vi "25-1.vi"() -> ()   [LabVIEW 2019, in "25.lvlib"]
uses:
  25.lvlib
panel:
  in  "Sample?":bool
  out "Array":u32[][](array[colorbox])
  out "Steps":i32
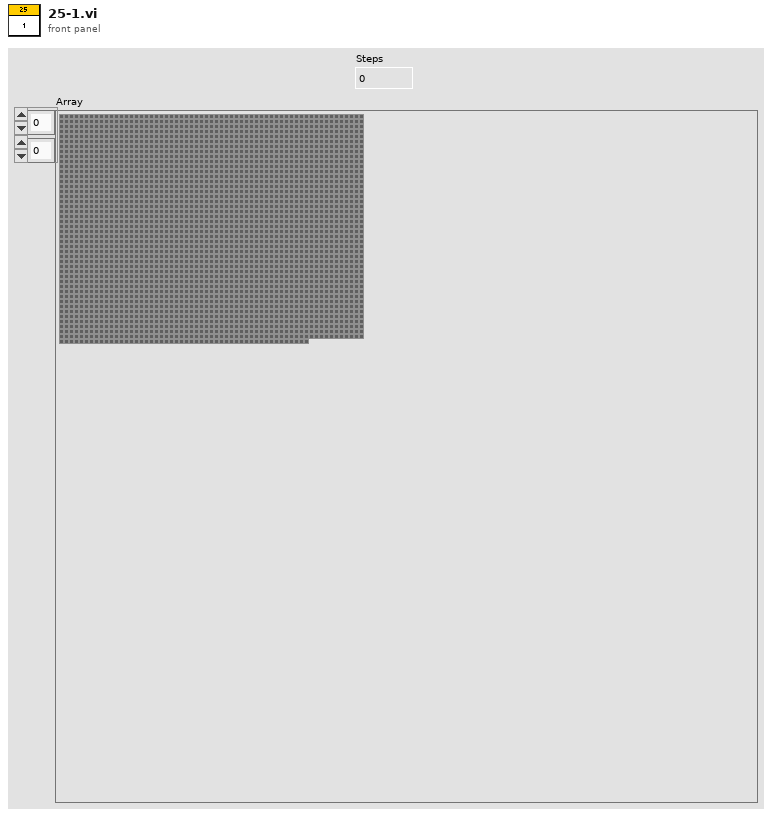
[diagram p1: front panel]
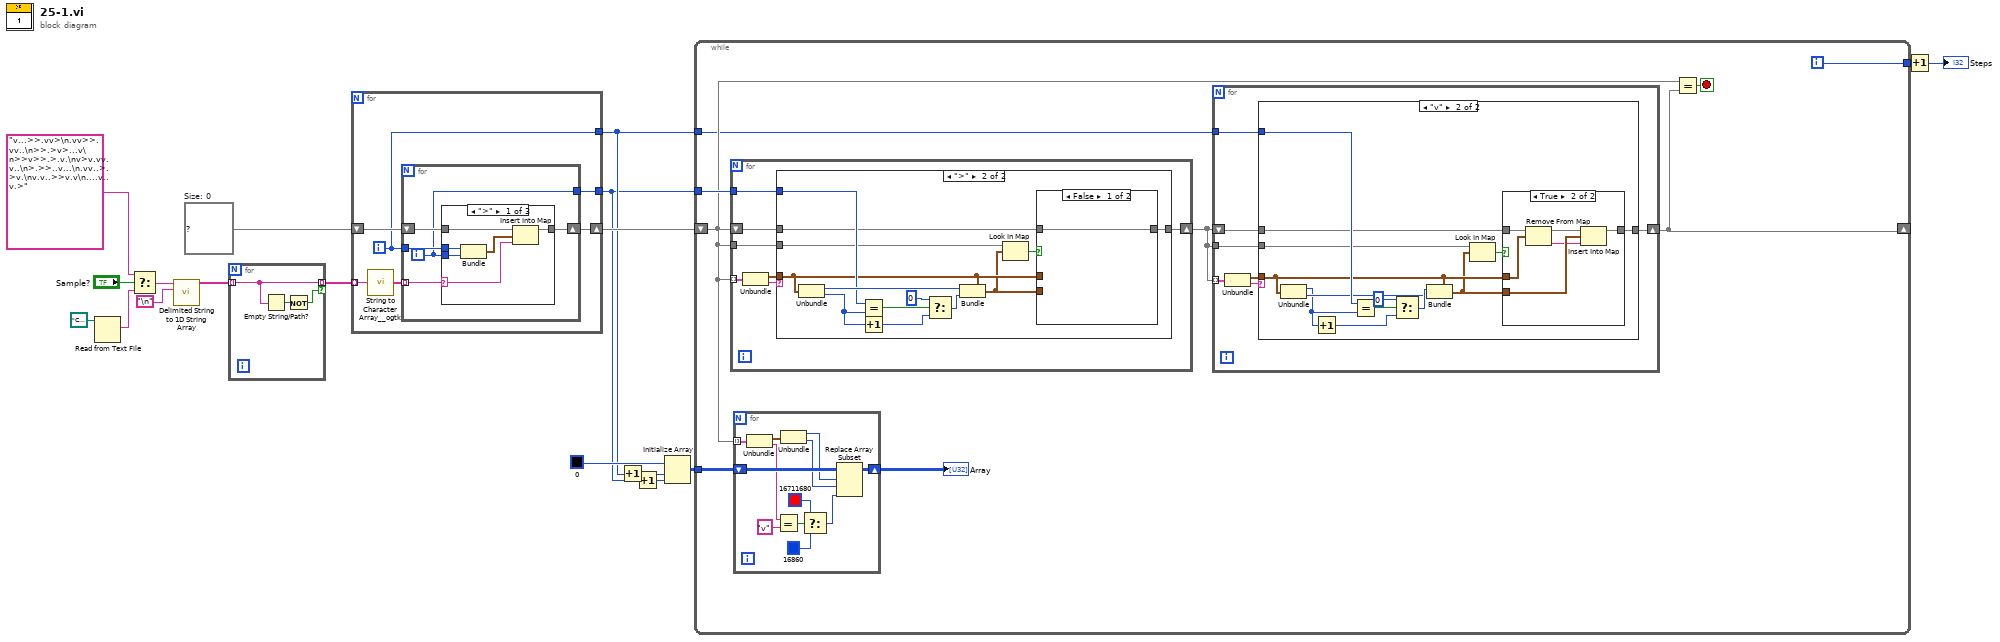
[diagram p0: block diagram]
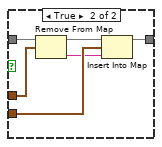
[diagram p5: hidden frame]
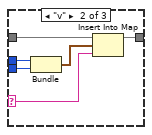
[diagram p6: hidden frame]
diagram:
  w17 = map{cluster{"Row":i32, "Column":i32}, string} {}  # Size: 0
  n1 = Read from Text File(file (use dialog)=path "C:/Users/craig.walker/Documents/GitHub/lv2019-Advent-of-Code-2021/25/input.txt") -> (text=w4:string)  [unwired: 3 in, 3 out]
  n2 = Select(t="v...>>.vv>\n.vv>>.vv..\n>>.>v>...v\n>>v>>.>.v.\nv>v.vv.v..\n>.>>..v...\n.vv..>.>v.\nv.v..>>v.v\n....v..v.>", s="Sample?", f=w4) -> (s? t:f=w6:string)
  n3 = call <vilib>:"Delimited String to 1D String Array.vi"("delimiter"="\n", "delimited string"=w6) -> ("string array"=w2:string[])  [unwired: 9 in]
  n4 = for {
    tunnel: w2 -> [w21] mode=indexing
    tunnel: [w21] -> w1 mode=indexing if=w19
    n5 = Empty String/Path?(string/path=w21) -> (empty?=w20:bool)
    n6 = Not(x=w20) -> (.not. x?=w19:bool)
  }
  n7 = for {
    tunnel: w1 -> [w27] mode=indexing
    shift-right: [w24] -> w16
    shift-left: w17 -> [w25]
    tunnel: [w23] -> w9
    tunnel: [w22] -> w8
    i -> [w23]
    n8 = call <userlib>:"String to Character Array__ogtk.vi"("Input String"=w27) -> ("Character Array"=w26:string[])
    n9 = for {
      tunnel: w26 -> [w32] mode=indexing
      shift-right: [w30] -> w24
      shift-left: w25 -> [w31]
      tunnel: w23 -> [w29]
      tunnel: [w28] -> w22
      i -> [w28]
      n10 = case shown="\">\"" w32 {
        selector: w32 -> [w33 w39 _]
        tunnel: w31 -> [w38 w44 w45]
        tunnel: [w37 w43 w45] -> w30
        tunnel: w29 -> [w35 w41 _]
        tunnel: w28 -> [w34 w40 _]
        frame ">" {
          n11 = Bundle(w35, w34) -> (w36:cluster{i32, i32})  [unwired: 1 in]
          n12 = Insert Into Map(map in=w38, key=w36, value=w33) -> (map out=w37:map{cluster{"Row":i32, "Column":i32}, string})  [unwired: 2 out]
        }
        frame "v" {
          n13 = Bundle(w41, w40) -> (w42:cluster{i32, i32})  [unwired: 1 in]
          n14 = Insert Into Map(map in=w44, key=w42, value=w39) -> (map out=w43:map{cluster{"Row":i32, "Column":i32}, string})  [unwired: 2 out]
        }
        frame Default {
        }
      }
    }
  }
  n15 = Increment(x=w9) -> (x+1=w11:i32)
  n16 = Increment(x=w8) -> (x+1=w10:i32)
  n17 = Initialize Array(u32 0, w11, w10) -> (w13:u32[][])
  n18 = while {
    shift-right: [w50] -> _
    shift-left: w16 -> [w47]
    tunnel: w8 -> [w54]
    tunnel: w9 -> [w46]
    tunnel: [w51] -> w15
    tunnel: w13 -> [w49]
    i -> [w51]
    stop <- w52 stop-if-true
    n19 = for {
      tunnel: w47 -> [w97] mode=indexing
      tunnel: w47 -> [w101]
      tunnel: w54 -> [w98]
      shift-right: [w95] -> w53
      shift-left: w47 -> [w96]
      n20 = Unbundle(w97) -> (w99:cluster{"Row":i32, "Column":i32}, "String"=w100:string)
      n21 = case shown="\">\"" w100 {
        tunnel: w101 -> [_ w109]
        tunnel: w99 -> [_ w106]
        tunnel: w98 -> [_ w114]
        tunnel: w96 -> [w102 w108]
        tunnel: [w102 w107] -> w95
        frame Default {
        }
        frame ">" {
          n22 = Unbundle(w106) -> ("Row"=w115:i32, "Column"=w103:i32)
          n23 = Equal?(x=w114, y=w103) -> (x = y?=w113:bool)
          n24 = Increment(x=w103) -> (x+1=w104:i32)
          n25 = Select(t=0, s=w113, f=w104) -> (s? t:f=w111:i32)
          n26 = Bundle(cluster=w106, "Row"=w115, "Column"=w111) -> (w105:cluster{"Row":i32, "Column":i32})
          n27 = Look In Map(map=w109, key=w105) -> (key not found?=w110:bool)  [unwired: 1 in, 1 out]
          n28 = case shown="False" w110 {
            tunnel: w108 -> [w116 w122]
            tunnel: [w116 w119] -> w107
            tunnel: w106 -> [_ w121]
            tunnel: w105 -> [_ w118]
            frame False {
            }
            frame True {
              n29 = Remove From Map(10:w121, 11:w122) -> (1:w117:string, 3:w120:map{cluster{"Row":i32, "Column":i32}, string})  [unwired: 1 out]
              n30 = Insert Into Map(map in=w120, key=w118, value=w117) -> (map out=w119:map{cluster{"Row":i32, "Column":i32}, string})  [unwired: 2 out]
            }
          }
        }
      }
    }
    n31 = for {
      tunnel: w47 -> [w65] mode=indexing
      shift-right: [w57] -> w48
      shift-left: w49 -> [w66]
      n32 = Unbundle(w65) -> (w64:cluster{"Row":i32, "Column":i32}, "String"=w61:string)
      n33 = Equal?(x=w61, y="v") -> (x = y?=w59:bool)
      n34 = Unbundle(w64) -> ("Row"=w63:i32, "Column"=w62:i32)
      n35 = Select(t=u32 16711680, s=w59, f=u32 16860) -> (s? t:f=w58:u32)
      n36 = Replace Array Subset(array=w66, new element=w58, index (row)=w63, index (col)=w62) -> (w57:u32[][])
    }
    "Array" <- w48
    n37 = for {
      tunnel: w53 -> [w69] mode=indexing
      tunnel: w53 -> [w73]
      tunnel: w46 -> [w70]
      shift-right: [w67] -> w50
      shift-left: w53 -> [w68]
      n38 = Unbundle(w69) -> (w71:cluster{"Row":i32, "Column":i32}, "String"=w72:string)
      n39 = case shown="\"v\"" w72 {
        tunnel: w73 -> [_ w83]
        tunnel: w71 -> [_ w80]
        tunnel: w70 -> [_ w87]
        tunnel: w68 -> [w74 w82]
        tunnel: [w74 w81] -> w67
        frame Default {
        }
        frame "v" {
          n40 = Unbundle(w80) -> ("Row"=w75:i32, "Column"=w77:i32)
          n41 = Increment(x=w75) -> (x+1=w76:i32)
          n42 = Equal?(x=w87, y=w75) -> (x = y?=w86:bool)
          n43 = Select(t=0, s=w86, f=w76) -> (s? t:f=w78:i32)
          n44 = Bundle(cluster=w80, "Row"=w78, "Column"=w77) -> (w79:cluster{"Row":i32, "Column":i32})
          n45 = Look In Map(map=w83, key=w79) -> (key not found?=w84:bool)  [unwired: 1 in, 1 out]
          n46 = case shown="True" w84 {
            tunnel: w82 -> [w88 w94]
            tunnel: [w88 w91] -> w81
            tunnel: w80 -> [_ w93]
            tunnel: w79 -> [_ w90]
            frame False {
            }
            frame True {
              n47 = Remove From Map(10:w93, 11:w94) -> (1:w89:string, 3:w92:map{cluster{"Row":i32, "Column":i32}, string})  [unwired: 1 out]
              n48 = Insert Into Map(map in=w92, key=w90, value=w89) -> (map out=w91:map{cluster{"Row":i32, "Column":i32}, string})  [unwired: 2 out]
            }
          }
        }
      }
    }
    n49 = Equal?(x=w47, y=w50) -> (x = y?=w52:bool)
  }
  n50 = Increment(x=w15) -> (x+1=→"Steps":i32)
